vi "PredetControlSequence (SubVI).vi"(1 "Predet Freq (Hz)":dbl=20.0 format="%#_13g", 3 "Error In":errorcluster) -> (10 "Error Out":errorcluster)   [LabVIEW 2016]
uses:
  <vilib>/DAQmx/write.llb/DAQmx Write (Digital 1D Wfm NChan NSamp).vi
  <resource>/objmgr/daqmx.rc
  <vilib>/DAQmx/create/channels.llb/DAQmx Create Channel (DO-Digital Output).vi
  <vilib>/DAQmx/configure/timing.llb/DAQmx Timing (Sample Clock).vi
panel:
  out "Digital Waveform Graph":digitalwaveform[](graph)
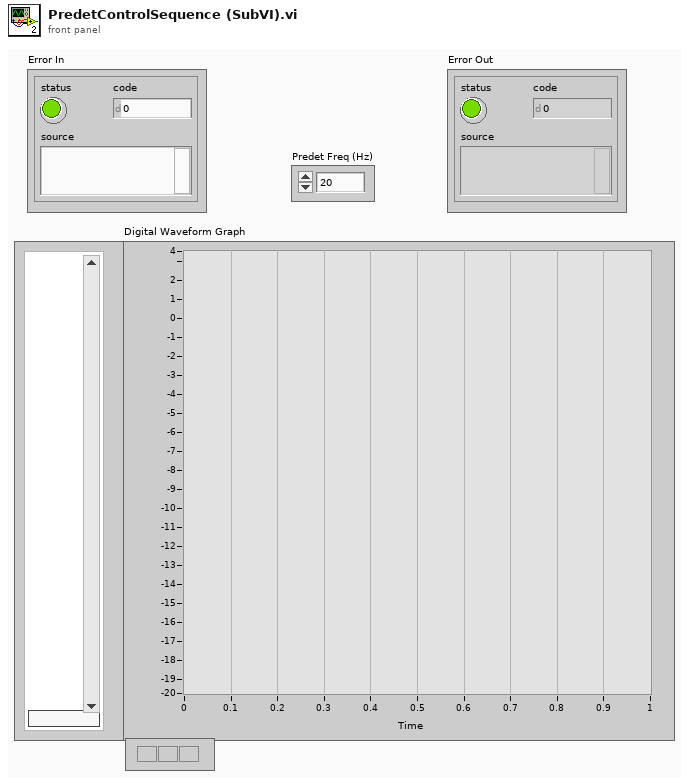
[diagram p1: front panel]
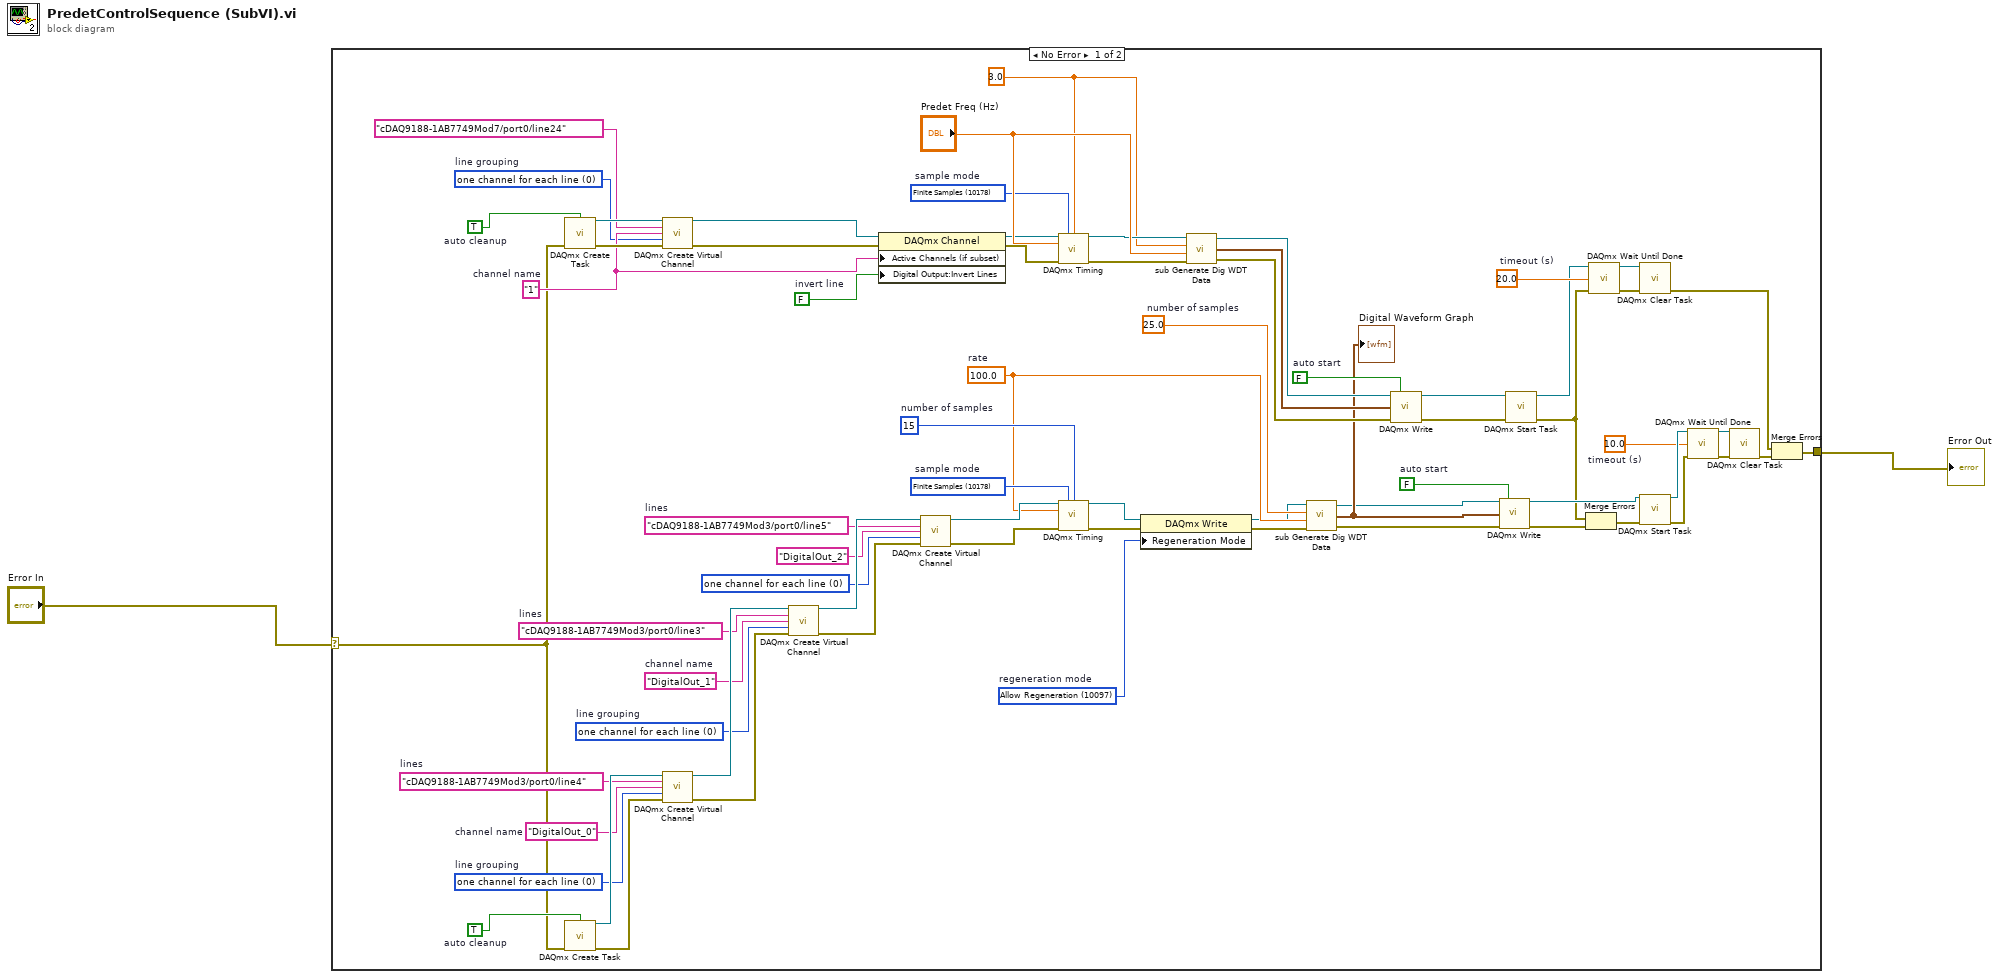
[diagram p0: block diagram]
diagram:
  n1 = case shown="No Error" "Error In" {
    selector: "Error In" -> [w3 w73]
    tunnel: [w4 w73] -> w2
    frame No Error {
      w17 = 10.0  # timeout (s)
      w23 = 20.0  # timeout (s)
      w40 = "cDAQ9188-1AB7749Mod3/port0/line5"  # lines
      w38 = 0 items=["one channel for each line", "one channel for all lines"] ("line grouping")
      w37 = 10097 items=["Allow Regeneration"=10097, "Do Not Allow Regeneration"=10158]  # regeneration mode
      w36 = 10178 items=["Finite Samples"=10178, "Continuous Samples"=10123, "Hardware Timed Single Point"=12522]  # sample mode
      w35 = 15  # number of samples
      w13 = 100.0  # rate
      w32 = 0 items=["one channel for each line", "one channel for all lines"]  # line grouping
      w33 = "DigitalOut_1"  # channel name
      w34 = "cDAQ9188-1AB7749Mod3/port0/line3"  # lines
      w29 = 0 items=["one channel for each line", "one channel for all lines"]  # line grouping
      w30 = "DigitalOut_0"  # channel name
      w31 = "cDAQ9188-1AB7749Mod3/port0/line4"  # lines
      w28 = TRUE  # auto cleanup
      w12 = 25.0  # number of samples
      w27 = FALSE  # auto start
      w59 = 3.0 ("number of samples")
      w60 = 10178 items=["Finite Samples"=10178, "Continuous Samples"=10123, "Hardware Timed Single Point"=12522]  # sample mode
      w55 = FALSE  # invert line
      w56 = 0 items=["one channel for each line", "one channel for all lines"]  # line grouping
      w57 = "1"  # channel name
      w54 = TRUE  # auto cleanup
      w53 = FALSE  # auto start
      n2 = call <vilib>:"DAQmx Create Task.vi"("auto cleanup"=w54, "error in"=w3) -> ("task out"=w67:refnum<k21>, "error out"=w68:errorcluster)  [unwired: 3 in, 9 out]
      n3 = call <vilib>:"DAQmx Create Task.vi"("auto cleanup"=w28, "error in"=w3) -> ("task out"=w42:refnum<k21>, "error out"=w41:errorcluster)  [unwired: 12 in]
      n4 = call-poly <vilib>:"DAQmx Create Virtual Channel.vi"("task in"=w67, "lines"=tag "cDAQ9188-1AB7749Mod7/port0/line24", "name to assign"=w57, "line grouping"=w56, "error in"=w68) -> ("task out"=w66:refnum<k21>, "error out"=w65:errorcluster)  [unwired: 9 out]
      n5 = call-poly <vilib>:"DAQmx Create Virtual Channel.vi"("task in"=w42, "lines"=w31, "name to assign"=w30, "line grouping"=w29, "error in"=w41) -> ("task out"=w44:refnum<k21>, "error out"=w43:errorcluster)  [unwired: 9 in]
      n6 = call-poly <vilib>:"DAQmx Create Virtual Channel.vi"("task in"=w44, "lines"=w34, "name to assign"=w33, "line grouping"=w32, "error in"=w43) -> ("task out"=w50:refnum<k21>, "error out"=w48:errorcluster)  [unwired: 9 in]
      n7 = property class="DAQmx Channel"(reference=w66, error in=w65, "Active Channels (if subset)"=w57, "Digital Output:Invert Lines"=w55) -> (reference out=w63:refnum<k21>, error out=w64:errorcluster)
      n8 = call-poly <vilib>:"DAQmx Create Virtual Channel.vi"("task in"=w50, "lines"=w40, "name to assign"="DigitalOut_2", "line grouping"=w38, "error in"=w48) -> ("task out"=w49:refnum<k21>, "error out"=w47:errorcluster)  [unwired: 9 in]
      n9 = call-poly <vilib>:"DAQmx Timing.vi"("task/channels in"=w63, "sample mode"=w60, "samples per channel"=w59, "rate"="Predet Freq (Hz)", "error in"=w64) -> ("task out"=w62:refnum<k21>, "error out"=w61:errorcluster)  [unwired: 2 in, 7 out]
      n10 = call-poly <vilib>:"DAQmx Timing.vi"("task/channels in"=w49, "sample mode"=w36, "samples per channel"=w35, "rate"=w13, "error in"=w47) -> ("task out"=w46:refnum<k21>, "error out"=w45:errorcluster)  [unwired: 9 in]
      n11 = property class="DAQmx Write"(reference=w46, error in=w45, "Regeneration Mode"=w37) -> (reference out=w9:refnum<k21>, error out=w14:errorcluster)
      n12 = call <vilib>:"sub Generate Dig WDT Data.vi"("task in"=w62, "number of samples"=w59, "update rate"="Predet Freq (Hz)", "error in"=w61) -> ("task out"=w70:refnum<k21>, "data"=w69:digitalwaveform[], "error out"=w71:errorcluster)  [unwired: 1 out]
      n13 = call <vilib>:"sub Generate Dig WDT Data.vi"("task in"=w9, "number of samples"=w12, "update rate"=w13, "error in"=w14) -> ("task out"=w8:refnum<k21>, "data"=w10:digitalwaveform[], "error out"=w11:errorcluster)  [unwired: 1 out]
      "Digital Waveform Graph" <- w10
      n14 = call-poly <vilib>:"DAQmx Write.vi"("task/channels in"=w70, "auto start"=w53, "data"=w69, "error in"=w71) -> ("task out"=w52:refnum<k21>, "error out"=w51:errorcluster)  [unwired: 10 out]
      n15 = call-poly <vilib>:"DAQmx Write.vi"("task/channels in"=w8, "auto start"=w27, "data"=w10, "error in"=w11) -> ("task out"=w26:refnum<k21>, "error out"=w16:errorcluster)  [unwired: 9 in, 1 out]
      n16 = call <vilib>:"DAQmx Start Task.vi"("task/channels in"=w52, "error in"=w51) -> ("task out"=w22:refnum<k21>, "error out"=w7:errorcluster)  [unwired: 12 out]
      n17 = Merge Errors(w7, w16) -> (w15:errorcluster)
      n18 = call <vilib>:"DAQmx Wait Until Done.vi"("task/channels in"=w22, "timeout (sec)"=w23, "error in"=w7) -> ("task out"=w24:refnum<k21>, "error out"=w25:errorcluster)  [unwired: 11 out]
      n19 = call <vilib>:"DAQmx Clear Task.vi"("task in"=w24, "error in"=w25) -> ("error out"=w5:errorcluster)  [unwired: 13 in]
      n20 = call <vilib>:"DAQmx Start Task.vi"("task/channels in"=w26, "error in"=w15) -> ("task out"=w21:refnum<k21>, "error out"=w20:errorcluster)  [unwired: 12 in]
      n21 = call <vilib>:"DAQmx Wait Until Done.vi"("task/channels in"=w21, "timeout (sec)"=w17, "error in"=w20) -> ("task out"=w18:refnum<k21>, "error out"=w19:errorcluster)  [unwired: 11 in]
      n22 = call <vilib>:"DAQmx Clear Task.vi"("task in"=w18, "error in"=w19) -> ("error out"=w6:errorcluster)  [unwired: 13 in]
      n23 = Merge Errors(w5, w6) -> (w4:errorcluster)
    }
    frame Error {
    }
  }
  "Error Out" <- w2
